vi "FormatThreadedCollect.vi"(2 "thread #":i32, 3 "collect":string) -> (0 "python object":string)   [LabVIEW 2014, in "Python Functions.lvlib"]
uses:
  Python Functions.lvlib
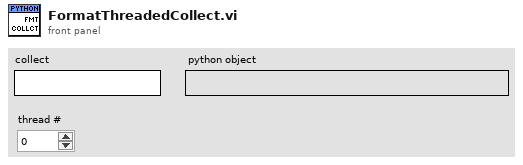
[diagram p1: front panel]
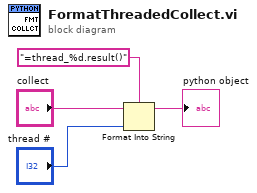
[diagram p0: block diagram]
diagram:
  n1 = Format Into String(format string="=thread_%d.result()", initial string="collect", "thread #") -> (resulting string=→"python object":string)  [unwired: 1 in, 1 out]
